vi "ReadFGV Err.vi"(8 "error in (no error)":errorcluster, 10 "0Cv/1ST":i32, 11 "Vision AI in":refnum<class "Vision AI.lvclass">) -> (0 "error out":errorcluster, 3 "Vision AI out":refnum<class "Vision AI.lvclass">)   [LabVIEW 2019, in "Vision AI.lvclass"]
uses:
  Vision AI.lvclass
  Ctrl/Auto Inspection Data Name.ctl
  Ctrl/Auto Inspection Station Name2.ctl
  f4bb030d-703d-4c2a-97ec-b4631f127a02.vi
  <vilib>/JDP Science/JSONtext/JSON text to Variant.vi
  FlowIOCtrl.lvclass
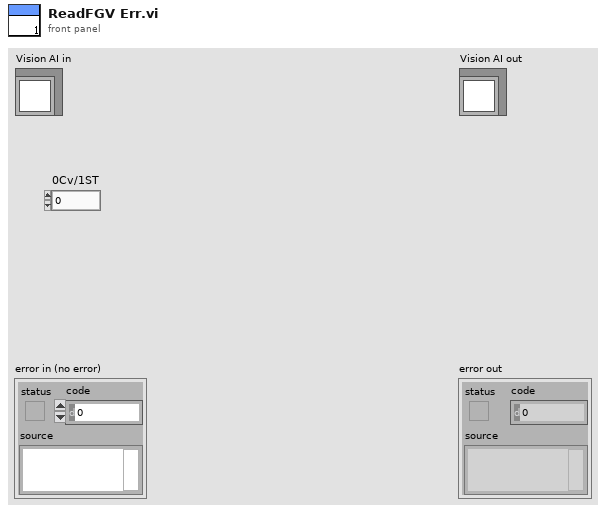
[diagram p1: front panel]
types:
  T1 = typedef "Auto Inspection Data Name.ctl" = enum16{"LocalRun", "ItemSN(TimeCode)", "CurrentAction", "Error", "Data", "OKNG", "電壓值", "電壓值判斷", "電流值", "電流值判斷", "Laser1 Data", "Laser2 Data", "Laser OKNG", "StationNO"}
  T2 = typedef "Auto Inspection Station Name2.ctl" = enum16{"S1Barcode", "S2Measure", "S3Measure", "S4Measure", "S5Measure", "S11_LaserCheck", "S8_Vision AI"}
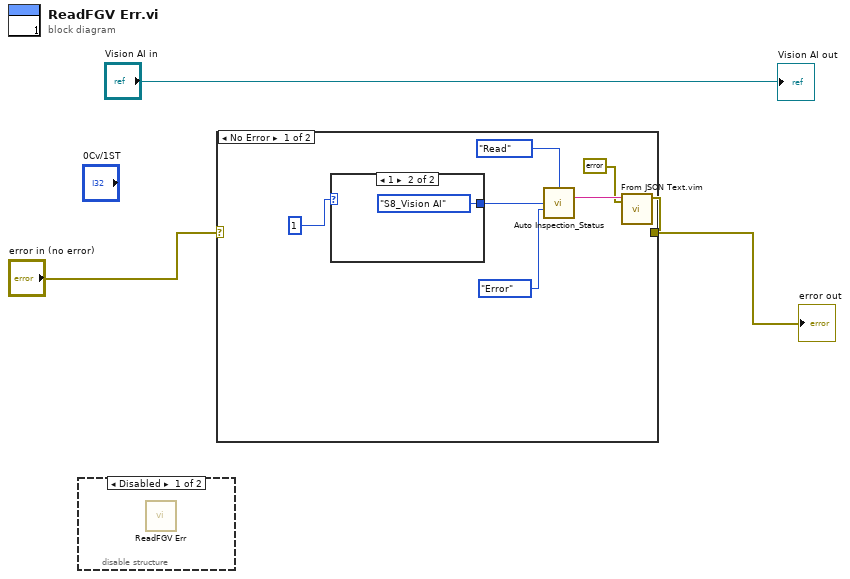
[diagram p0: block diagram]
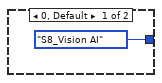
[diagram p2: hidden frame]
diagram:
  n1 = disable-structure shown="Disabled" {
    frame Disabled {
      n2 = call-parent "ReadFGV Err.vi"() -> ()  [unwired: 10 in, 2 out]
    }
    frame Enabled {
    }
  }
  n3 = case shown="No Error" "error in (no error)" {
    selector: "error in (no error)" -> [_ w13]
    tunnel: [w5 w13] -> w1
    frame No Error {
      n4 = case shown="1" 1 {
        tunnel: [Auto_Inspection_Station_Name2."S8_Vision AI" ("Station") Auto_Inspection_Station_Name2."S8_Vision AI" ("Station")] -> w9
        frame 0, Default {
        }
        frame 1 {
        }
      }
      n5 = call "Auto Inspection_Status.vi"("Action"=enum16{"Initial", "Write", "Read"}."Read", "Station"=w9, "Data"=Auto_Inspection_Data_Name."Error") -> ("DataOut"=w7:string)  [unwired: 10 in, 2 out]
      n6 = call "From JSON Text.vim"("Data Type and Default Value"=errorcluster {"status"=FALSE, "code"=0, "source"=""} ("error constant"), "JSON"=w7) -> ("Data out"=w5:errorcluster)  [unwired: 8 in, 1 out]
    }
    frame Error {
    }
  }
  "error out" <- w1
  "Vision AI out" <- "Vision AI in"
